vi "AlazarGetMaxRecordsCapable.vi"(0 "Handle":u64, 11 "error in (no error)":errorcluster) -> (4 "Handle":u64, 6 "Samples Per Record":u32, 8 "Max Records Per Capture":u32, 10 "Return Code":u32, 15 "error out":errorcluster)   [LabVIEW 2009]
doc: "Calculate the maximum number of records that can be captured to on-board memory given the requested number of samples per record."
uses:
  ATSApi.dll
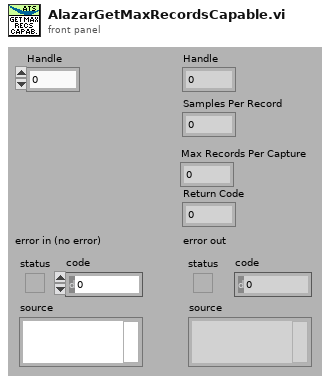
[diagram p1: front panel]
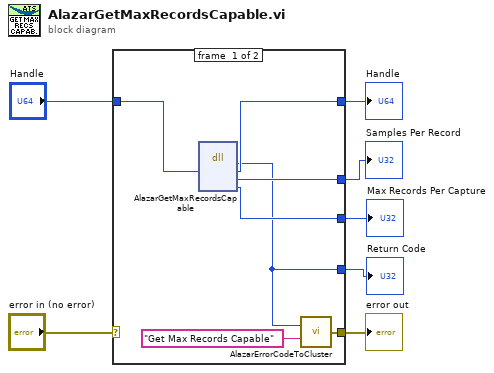
[diagram p0: block diagram]
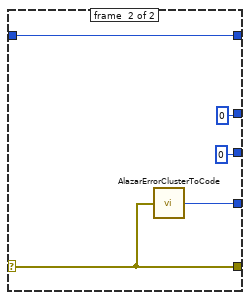
[diagram p2: hidden frame]
diagram:
  n1 = case shown="No Error" "error in (no error)" {
    selector: "error in (no error)" -> [_ w19]
    tunnel: [w10 w19] -> w6
    tunnel: [w9 w18] -> w5
    tunnel: "Handle" -> [w14 w17]
    tunnel: [w13 w17] -> w3
    tunnel: [w12 u32 0] -> w2
    tunnel: [w11 u32 0] -> w1
    frame #0 {
      n2 = dll-call lib="ATSApi.dll" fn="AlazarGetMaxRecordsCapable"("handle"=w14) -> ("return type"=w9:u32, "handle"=w13:u64, "samplesPerRecord"=w12:u32, "maxRecordsPerCapture"=w11:u32)  [unwired: 5 in, 2 out]
      n3 = call "AlazarErrorCodeToCluster.vi"("Message"="Get Max Records Capable", "Error Code"=w9) -> ("error out"=w10:errorcluster)
    }
    frame #1 {
      n4 = call "AlazarErrorClusterToCode.vi"("error in (no error)"=w19) -> ("Error Code"=w18:u32)
    }
  }
  "Handle" <- w3
  "error out" <- w6
  "Return Code" <- w5
  "Samples Per Record" <- w2
  "Max Records Per Capture" <- w1
